vi "Remove Duplicates from TSM Pin Information Array.vi"(0 "Pins and/or Pin Groups Information":T3[](array[typedef]), 5 "Expanded Pin Information in":T1[](array[typedef])) -> (6 "De-Duped Expanded Pin Information out":T1[](array[typedef]))   [LabVIEW 2020]
uses:
  TSM Expanded Pin Information.ctl
  TSM Pin Type Identifier.ctl
  TSM Pin Information.ctl
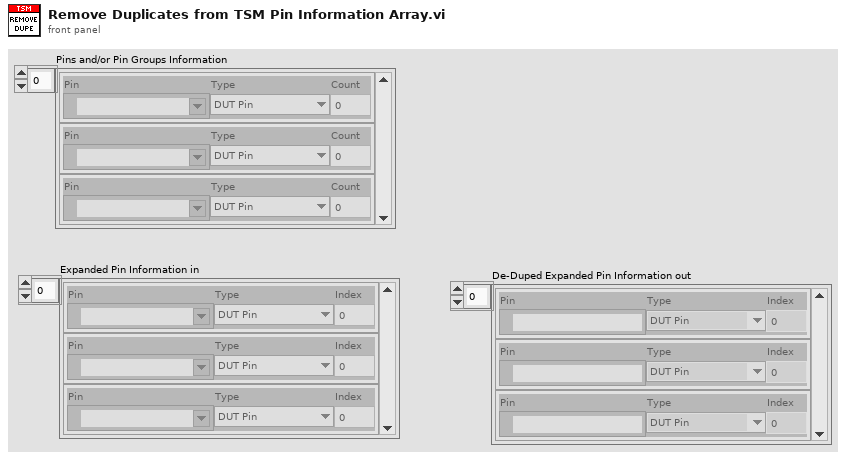
[diagram p1: front panel]
types:
  T1 = typedef "TSM Expanded Pin Information.ctl" = cluster{"Pin":tag, "Type":T2, "Index":i32}
  T2 = typedef "TSM Pin Type Identifier.ctl" = enum8{"DUT Pin", "System Pin", "Pin Group", "Not Determined"}
  T3 = typedef "TSM Pin Information.ctl" = cluster{"Pin":tag, "Type":T2, "Count":i32}
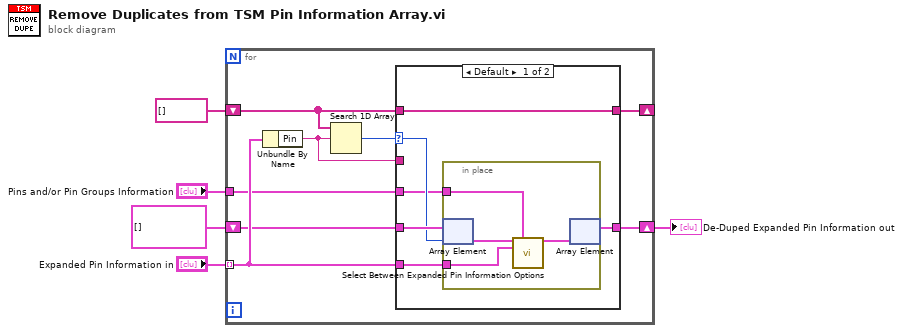
[diagram p0: block diagram]
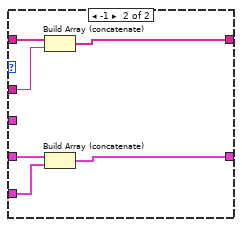
[diagram p2: hidden frame]
diagram:
  n1 = for {
    tunnel: "Expanded Pin Information in" -> [w9] mode=indexing
    shift-right: [w13] -> _
    shift-left: string[] [] -> [w10]
    shift-right: [w7] -> w1
    shift-left: T1[] [] ("Array") -> [w8]
    tunnel: "Pins and/or Pin Groups Information" -> [w6]
    n2 = Unbundle By Name(w9) -> ("Pin"=w12:tag)
    n3 = Search 1D Array(1D array=w10, element=w12) -> (index of element=w11:i32)  [unwired: 1 in]
    n4 = case shown="Default" w11 {
      selector: w11 -> [w16 _]
      tunnel: [w18 w29] -> w13
      tunnel: w12 -> [_ w28]
      tunnel: w10 -> [w18 w27]
      tunnel: w9 -> [w19 w25]
      tunnel: w8 -> [w17 w26]
      tunnel: [w15 w24] -> w7
      tunnel: w6 -> [w14 _]
      frame Default {
        n5 = in-place {
          in-place-border: w19 -> [w22]
          in-place-border: w14 -> [w20]
          n6 = in-place-array #1(w17, w16) -> (w23:T1)
          n7 = call "Select Between Expanded Pin Information Options.vi"("Current"=w23, "Pins and/or Pin Groups Information"=w20, "Duplicate"=w22) -> ("Best Choice Out"=w21:T1)  [unwired: 12 in]
          n8 = in-place-array #1(w21) -> (w15:T1[])  [unwired: 1 out]
        }
      }
      frame -1 {
        n9 = Build Array (concatenate)(w27, w28) -> (w29:string[])
        n10 = Build Array (concatenate)(w26, w25) -> (w24:T1[])
      }
    }
  }
  "De-Duped Expanded Pin Information out" <- w1
